vi "Event Handler.vi"(8 "error in (no error)":errorcluster, 10 "Stop Event Handler":refnum<user-event>, 11 "OrderSelection in":refnum<class "OrderSelection.lvclass">) -> (0 "error out":errorcluster)   [LabVIEW 2015, in "OrderSelection.lvclass"]
doc: "The <b>Event Handler VI</b> is a dynamic dispatch VI that should be overwritten if events are needed to create the enhanced QControl. \n\nBy inheriting from the main Control.lvclass the overwritten <b>Event Handler VI</b> will be launched asynchronously in the initialization of the QControl.\n<b> </b> <b> </b>\n©2016 Q Software Innovations, LLC (QSI)\nwritten by Quentin Alldredge\nproduced in LabVIEW 2015\n\nsupport@qsoftwareinnovations.com\nwww.qsoftwareinnovations.com\n\nAll rights reserved.\n\nRedistribution and use in source and binary forms, with or without modification, are permitted provided that the following conditions are met:\n\n * Redistributions of source code must retain the above copyright notice, this list of conditions and the following disclaimer.\n * Redistributions in binary form must reproduce the above copyright notice, this list of conditions and the following disclaimer in the documentation and/or other materials provided with the distribution.\n * Neither the name of Q Software Innovations, LLC. nor the names of its contributors may be used to endorse or promote products derived from this software without specific prior written permission.\n\nTHIS SOFTWARE IS PROVIDED BY THE COPYRIGHT HOLDERS AND CONTRIBUTORS \"AS IS\" AND ANY EXPRESS OR IMPLIED WARRANTIES, INCLUDING, BUT NOT LIMITED TO, THE IMPLIED WARRANTIES OF MERCHANTABILITY AND FITNESS FOR A PARTICULAR PURPOSE ARE DISCLAIMED. IN NO EVENT SHALL THE COPYRIGHT OWNER OR CONTRIBUTORS BE LIABLE FOR ANY DIRECT, INDIRECT, INCIDENTAL, SPECIAL, EXEMPLARY, OR CONSEQUENTIAL DAMAGES (INCLUDING, BUT NOT LIMITED TO, PROCUREMENT OF SUBSTITUTE GOODS OR SERVICES; LOSS OF USE, DATA, OR PROFITS; OR BUSINESS INTERRUPTION) HOWEVER CAUSED AND ON ANY THEORY OF LIABILITY, WHETHER IN CONTRACT, STRICT LIABILITY, OR TORT (INCLUDING NEGLIGENCE OR OTHERWISE) ARISING IN ANY WAY OUT OF THE USE OF THIS SOFTWARE, EVEN IF ADVISED OF THE POSSIBILITY OF SUCH DAMAGE."
uses:
  OrderSelection.lvclass
  <vilib>/Utility/miscctls.llb/LVPointTypeDef.ctl
  OrderSelection.lvclass/OrderSelection.ctl
  Write SelectedItem.vi
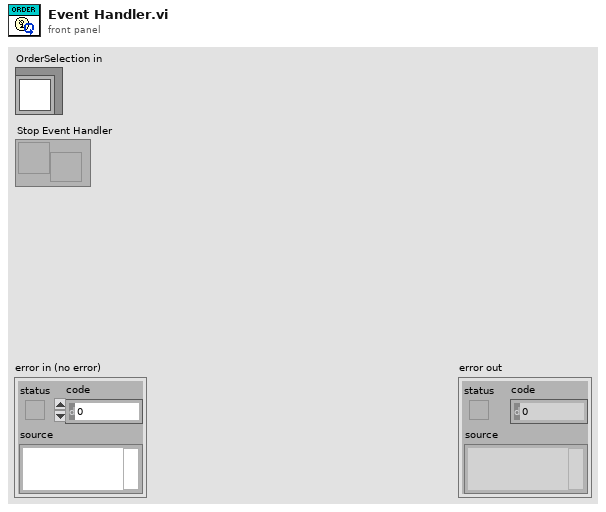
[diagram p1: front panel]
types:
  T1 = typedef "LVPointTypeDef.ctl" = cluster{"Horizontal":i16, "Vertical":i16}
  T2 = typedef "LVPoint32TypeDef.ctl" = cluster{"Horizontal":i32, "Vertical":i32}
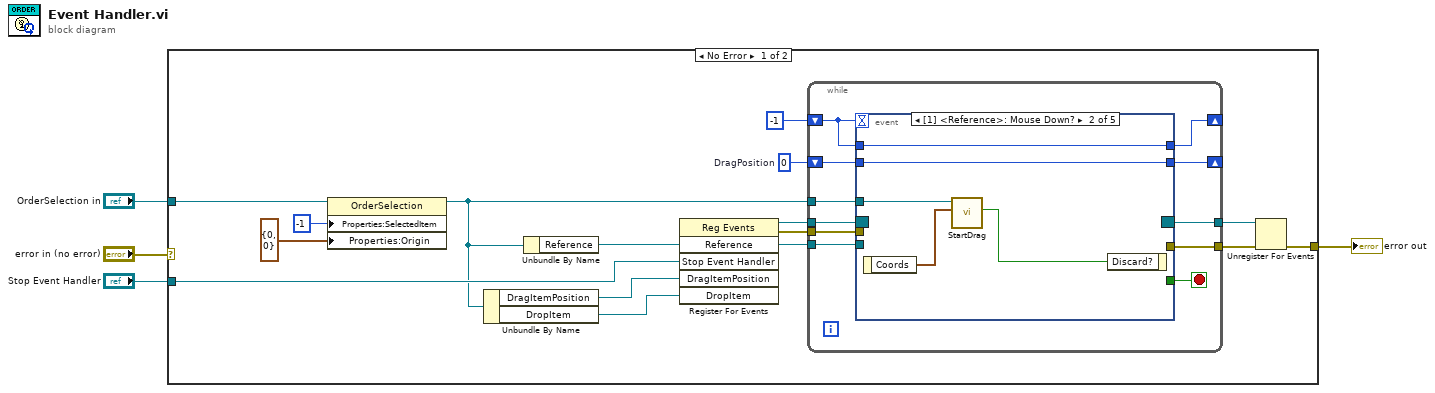
[diagram p0: block diagram]
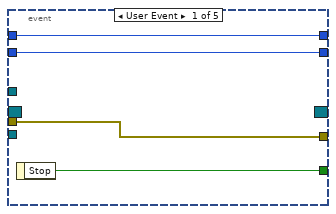
[diagram p2: hidden frame]
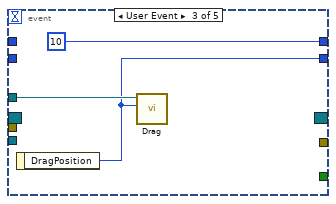
[diagram p3: hidden frame]
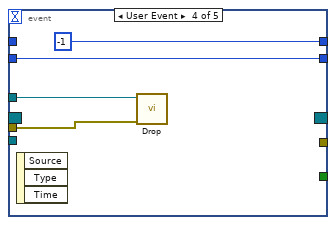
[diagram p4: hidden frame]
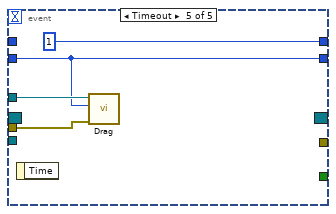
[diagram p5: hidden frame]
diagram:
  n1 = case shown="No Error" "error in (no error)" {
    selector: "error in (no error)" -> [_ w51]
    tunnel: [w6 w51] -> w3
    tunnel: "OrderSelection in" -> [w13 _]
    tunnel: "Stop Event Handler" -> [w14 _]
    frame No Error {
      w10 = 0  # DragPosition
      n2 = property class="OrderSelection"(reference=w13, "Properties:SelectedItem"=-1 ("SelectedItem"), "Properties:Origin"=T1 {"Horizontal"=0, "Vertical"=0} ("Origin: All Elements")) -> (reference out=w5:refnum<class "OrderSelection.lvclass">)  [unwired: 1 in, 1 out]
      n3 = Unbundle By Name(w5) -> ("DragItemPosition"=w7:refnum<user-event>, "DropItem"=w8:refnum<user-event>)
      n4 = Unbundle By Name(w5) -> ("Reference"=w15:refnum<vi>)
      n5 = register-events(w15, w14, w7, w8) -> (reference out=w19:refnum<event-registration>, error out=w18:errorcluster)  [unwired: 2 in]
      n6 = while {
        tunnel: w19 -> [w30]
        tunnel: w18 -> [w28]
        tunnel: [w27] -> w17
        tunnel: [w25] -> w16
        tunnel: w15 -> [w24]
        tunnel: w5 -> [w29]
        shift-right: [w22] -> _
        shift-left: -1 -> [w23]
        shift-right: [w21] -> _
        shift-left: w10 -> [w20]
        stop <- w26 stop-if-true
        n7 = event shown="[1] <Reference>: Mouse Down?" {
          selector: w30 -> [_ _ _ _ _]
          dyn-events: [_ _ _ _ _] -> w25
          timeout: w23 -> [_ _ _ _ _]
          tunnel: w29 -> [_ w39 w42 w46 w50]
          tunnel: w28 -> [w34 _ _ w45 w49]
          tunnel: [w34 _ _ _ _] -> w27
          tunnel: [w33 _ _ _ _] -> w26
          tunnel: w24 -> [_ _ _ _ _]
          tunnel: w23 -> [w32 w35 _ _ _]
          tunnel: [w32 w35 10 -1 1] -> w22
          tunnel: [w31 w36 w41 w43 w48] -> w21
          tunnel: w20 -> [w31 w36 _ w43 w48]
          event User Event {
            n8 = event-data() -> ("Stop"=w33:bool)  [unwired: 1 in]
          }
          event Mouse Down? {
            n9 = event-data() -> ("Coords"=w38:T2)  [unwired: 1 in]
            n10 = call "StartDrag.vi"("Coords"=w38, "OrderSelection in"=w39) -> ("InItem?"=w37:bool)  [unwired: 7 in, 2 out]
            n11 = event-data("Discard?"=w37) -> ()  [unwired: 1 in, 1 out]
          }
          event User Event {
            n12 = event-data() -> ("DragPosition"=w41:i32)  [unwired: 1 in]
            n13 = call "Drag.vi"("DragPosition"=w41, "OrderSelection in"=w42) -> ()  [unwired: 8 in, 2 out]
          }
          event User Event {
            n14 = event-data() -> ()  [unwired: 1 in, 3 out]
            n15 = call "Drop.vi"("error in (no error)"=w45, "OrderSelection in"=w46) -> ()  [unwired: 8 in, 2 out]
          }
          event Timeout {
            n16 = event-data() -> ()  [unwired: 1 in, 1 out]
            n17 = call "Drag.vi"("error in (no error)"=w49, "DragPosition"=w48, "OrderSelection in"=w50) -> ()  [unwired: 7 in, 2 out]
          }
        }
      }
      n18 = Unregister For Events(event registration refnum=w16, error in=w17) -> (error out=w6:errorcluster)
    }
    frame Error {
    }
  }
  "error out" <- w3
